vi "LVFunction_Imop_Get Sequence Size.vi"(0 "path":path, 11 "error in (no error)":errorcluster) -> (4 "path (dup)":path, 6 "Sizetab":u32, 15 "error out":errorcluster)   [LabVIEW 2020]
doc: "Get the size of the HasoData array from file.\n\n--------------------------------------------------------------------------------\n\n<B>sequence_file_pathIn</B> : Absolute path to sequence file.\n\n<B>sequence_file_pathOut</B> : Absolute path to sequence file.\n\n<B>sequence_size</B> : Sequence length (number of HasoData).\n\n<B>ErrorIn</B> : Error\n\n<B>ErrorOut</B> : Error"
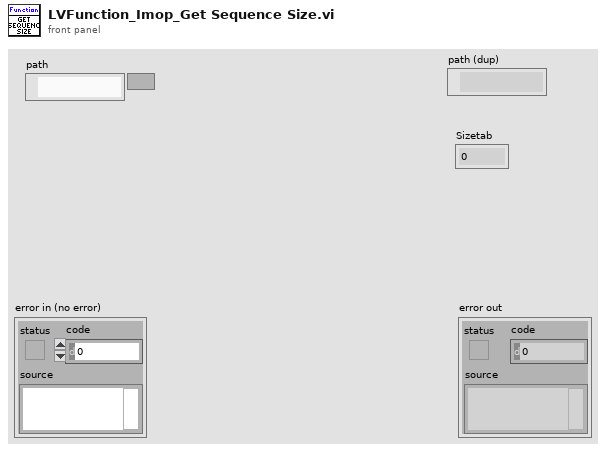
[diagram p1: front panel]
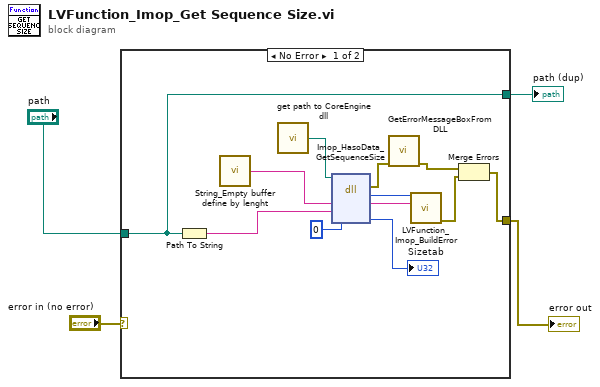
[diagram p0: block diagram]
diagram:
  n1 = case shown="No Error" "error in (no error)" {
    selector: "error in (no error)" -> [_ w18]
    tunnel: [w6 w18] -> w3
    tunnel: [w5 w17] -> w2
    tunnel: "path" -> [w5 w17]
    frame No Error {
      n2 = Path To String(path=w5) -> (string=w10:string)
      n3 = call "String_Empty buffer define by lenght.vi"() -> ("Empty buffer"=w14:string)  [unwired: 1 in]
      n4 = call "get path to CoreEngine dll.vi"() -> ("path to wavekit library"=w13:path)  [unwired: 14 in, 1 out]
      n5 = dll-call lib="D:/2_trunk/Soft_haso/ImOpCoreEngine4_LV2011/DLLs/ImopEngine4_vc100.dll" fn="Imop_HasoData_GetSequenceSize"(path in=w13, "message"=w14, "SequenceFilePath"=w10, "Sizetab"=u32 0) -> (error out=w12:errorcluster, "return type"=w16:i32, "message"=w15:string, "Sizetab"=→"Sizetab":u32)  [unwired: 3 in, 1 out]
      n6 = call "GetErrorMessageBoxFromDLL.vi"("error IN"=w12) -> ("error OUT"=w8:errorcluster)  [unwired: 10 in]
      n7 = call "LVFunction_Imop_BuildError.vi"("code"=w16, "String to Prepend to source (\"\")"=w15) -> ("error out"=w7:errorcluster)  [unwired: 13 in]
      n8 = Merge Errors(w8, w7) -> (w6:errorcluster)
    }
    frame Error {
    }
  }
  "error out" <- w3
  "path (dup)" <- w2
